vi "sm.main-shortest.vi"(10 "destination":fxp<+/-,32,2>, 11 "origin":fxp<+/-,32,2>) -> (3 "forward?":bool)   [LabVIEW 2019]
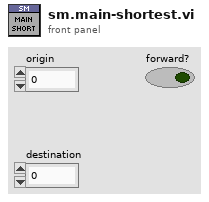
[diagram p1: front panel]
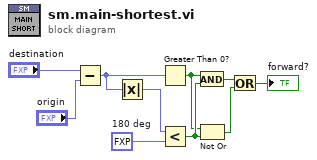
[diagram p0: block diagram]
diagram:
  w3 = fxp<+,1,0> 0.5  # 180 deg
  n1 = Subtract(x="destination", y="origin") -> (x-y=w4:fxp<+/-,33,3>)
  n2 = Absolute Value(x=w4) -> (abs(x)=w5:fxp<+,32,2>)
  n3 = Greater Than 0?(x=w4) -> (x > 0?=w7:bool)
  n4 = Less?(x=w5, y=w3) -> (x < y?=w8:bool)
  n5 = And(x=w7, y=w8) -> (x .and. y?=w6:bool)
  n6 = Not Or(1:w8, 2:w7) -> (0:w9:bool)
  n7 = Or(x=w6, y=w9) -> (x .or. y?=→"forward?":bool)
